vi "FPGA Tri Phase Sine Generator (FPGA).vi"() -> ()   [LabVIEW 2017]
uses:
  <vilib>/rvi/Arithmetic/AddSubMult/XNode/nirviSatArithmetic.xnode
  <vilib>/eio/EIONode/EIONode.xnode
panel:
  in  "initialize":bool
  in  "Sinewave Props 2":T1={"Phase Increment"=0, "Phase Offset"=0, "Scale Factor"=32767, "Amplitude Offset"=0}
  in  "Sinewave Props 1":T1={"Phase Increment"=0, "Phase Offset"=0, "Scale Factor"=32767, "Amplitude Offset"=0}
  in  "Sinewave Props 0":T1={"Phase Increment"=0, "Phase Offset"=0, "Scale Factor"=32767, "Amplitude Offset"=0}
  out "Sampling Rate Acheived?":bool
  out "Actual Loop Rate":u32
  in  "stop":bool
  in  "Desired Loop Rate (Ticks)":u32=2666666 caption="Update Interval (Ticks)"
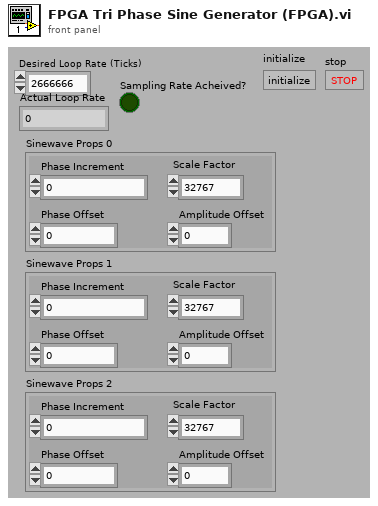
[diagram p1: front panel]
types:
  T1 = cluster{"Phase Increment":u32, "Phase Offset":u32, "Scale Factor":i16, "Amplitude Offset":i16}
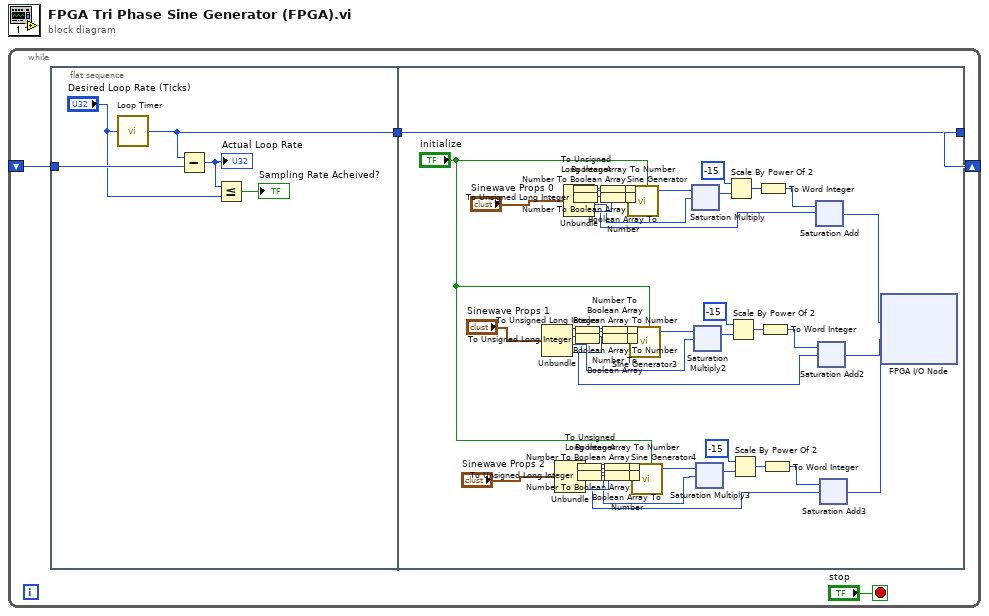
[diagram p0: block diagram]
diagram:
  n1 = while {
    shift-right: [w2] -> _
    shift-left: _ -> [w3]
    stop <- "stop" stop-if-true
    n2 = flat-sequence {
      tunnel: w3 -> [w9]
      tunnel: [w8] -> w1
      tunnel: [w60] -> w2
      tunnel: w1 -> [w60]
      frame #0 {
        n3 = call "Loop Timer"("Count(Ticks)"="Desired Loop Rate (Ticks)") -> ("Tick Count(Ticks)"=w8:u32)
        n4 = Subtract(x=w8, y=w9) -> (x-y=w7:u32)
        "Actual Loop Rate" <- w7
        n5 = Less Or Equal?(x=w7, y="Desired Loop Rate (Ticks)") -> (x <= y?=→"Sampling Rate Acheived?":bool)
      }
      frame #1 {
        n6 = Unbundle("Sinewave Props 1") -> ("Phase Increment"=w35:u32, "Phase Offset"=w36:u32, "Scale Factor"=w37:i16, "Amplitude Offset"=w38:i16)
        n7 = Unbundle("Sinewave Props 2") -> ("Phase Increment"=w34:u32, "Phase Offset"=w33:u32, "Scale Factor"=w32:i16, "Amplitude Offset"=w31:i16)
        n8 = Unbundle("Sinewave Props 0") -> ("Phase Increment"=w42:u32, "Phase Offset"=w41:u32, "Scale Factor"=w40:i16, "Amplitude Offset"=w39:i16)
        n9 = To Unsigned Long Integer(number=w42) -> (unsigned 32bit integer=w15:u32)
        n10 = To Unsigned Long Integer(number=w41) -> (unsigned 32bit integer=w12:u32)
        n11 = To Unsigned Long Integer(number=w35) -> (unsigned 32bit integer=w21:u32)
        n12 = To Unsigned Long Integer(number=w36) -> (unsigned 32bit integer=w18:u32)
        n13 = To Unsigned Long Integer(number=w34) -> (unsigned 32bit integer=w27:u32)
        n14 = To Unsigned Long Integer(number=w33) -> (unsigned 32bit integer=w24:u32)
        n15 = Number To Boolean Array(number=w15) -> (Boolean array=w13:bool[])
        n16 = Number To Boolean Array(number=w12) -> (Boolean array=w10:bool[])
        n17 = Number To Boolean Array(number=w21) -> (Boolean array=w19:bool[])
        n18 = Number To Boolean Array(number=w18) -> (Boolean array=w16:bool[])
        n19 = Number To Boolean Array(number=w27) -> (Boolean array=w25:bool[])
        n20 = Number To Boolean Array(number=w24) -> (Boolean array=w22:bool[])
        n21 = Boolean Array To Number(Boolean array=w13) -> (number=w14:fxp<+,32,0>)
        n22 = Boolean Array To Number(Boolean array=w10) -> (number=w11:fxp<+,32,0>)
        n23 = Boolean Array To Number(Boolean array=w19) -> (number=w20:fxp<+,32,0>)
        n24 = Boolean Array To Number(Boolean array=w16) -> (number=w17:fxp<+,32,0>)
        n25 = Boolean Array To Number(Boolean array=w25) -> (number=w26:fxp<+,32,0>)
        n26 = Boolean Array To Number(Boolean array=w22) -> (number=w23:fxp<+,32,0>)
        n27 = call "Sine Generator"("frequency (periods/tick)"=w14, "reset"="initialize", "phase offset (periods)"=w11) -> ("sine out"=w59:i16)  [unwired: 12 in]
        n28 = call "Sine Generator3"("frequency (periods/tick)"=w20, "reset"="initialize", "phase offset (periods)"=w17) -> ("sine out"=w53:i16)  [unwired: 12 in]
        n29 = call "Sine Generator4"("frequency (periods/tick)"=w26, "reset"="initialize", "phase offset (periods)"=w23) -> ("sine out"=w48:i16)  [unwired: 12 in]
        n30 = xnode ("Saturation Multiply")("x"=w59, "y"=w40) -> ("x*y"=w62:i32)
        n31 = xnode ("Saturation Multiply2")("x"=w53, "y"=w37) -> ("x*y"=w51:i32)
        n32 = xnode ("Saturation Multiply3")("x"=w48, "y"=w32) -> ("x*y"=w50:i32)
        n33 = Scale By Power Of 2(n=-15, x=w62) -> (x*2^n=w57:i32)
        n34 = Scale By Power Of 2(n=-15, x=w51) -> (x*2^n=w54:i32)
        n35 = Scale By Power Of 2(n=-15, x=w50) -> (x*2^n=w47:i32)
        n36 = To Word Integer(number=w57) -> (16bit integer=w56:i16)
        n37 = To Word Integer(number=w54) -> (16bit integer=w55:i16)
        n38 = To Word Integer(number=w47) -> (16bit integer=w46:i16)
        n39 = xnode ("Saturation Add")("x"=w56, "y"=w39) -> ("x+y"=w58:i16)
        n40 = xnode ("Saturation Add2")("x"=w55, "y"=w38) -> ("x+y"=w29:i16)
        n41 = xnode ("Saturation Add3")("x"=w46, "y"=w31) -> ("x+y"=w28:i16)
        n42 = xnode "FPGA I/O Node"("AO0"=w58, "AO1"=w29, "AO2"=w28) -> ()  [unwired: 3 in, 3 out]
      }
    }
  }
